vi "example 14 - splitters.vi"() -> ()   [LabVIEW 2020]
uses:
  ui-testing/ui-testing.lvlib
panel:
  out "Button clicked":string
  in  "A":bool
  in  "B":bool
  in  "C":bool
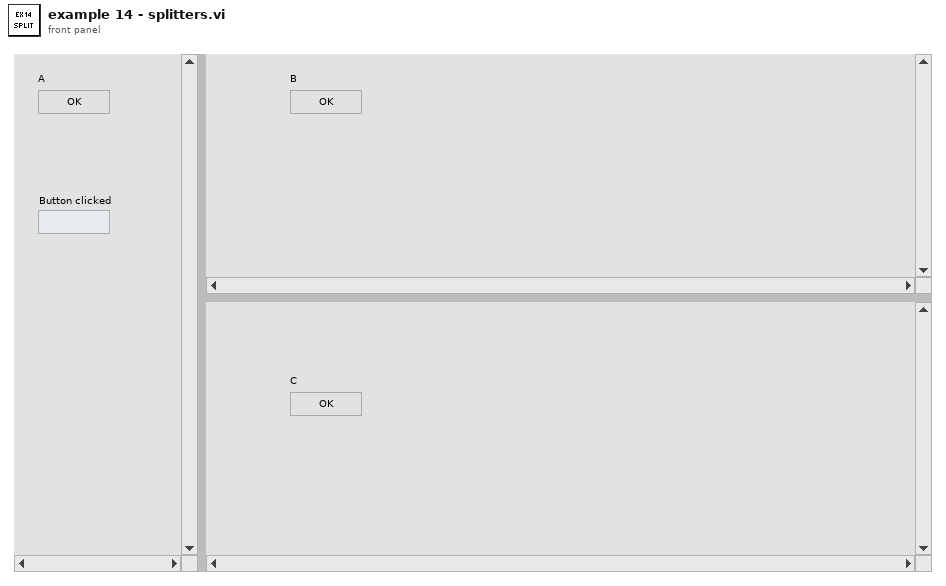
[diagram p1: front panel]
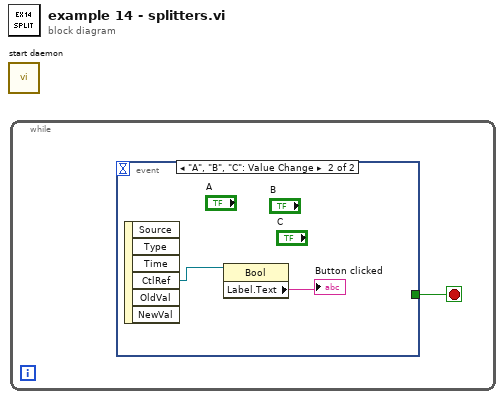
[diagram p0: block diagram]
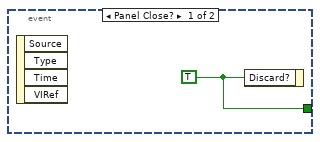
[diagram p2: hidden frame]
diagram:
  n1 = call "start daemon.vi"() -> ()  [unwired: 11 in, 1 out]
  n2 = while {
    stop <- w1 stop-if-true
    n3 = event shown="[1] \"A\", \"B\", \"C\": Value Change" {
      selector: _ -> [_ _]
      dyn-events: _ -> [_ _]
      timeout: _ -> [_ _]
      tunnel: [w2 _] -> w1
      event Panel Close? {
        w2 = TRUE
        n4 = event-data() -> ()  [unwired: 1 in, 4 out]
        n5 = event-data("Discard?"=w2) -> ()  [unwired: 1 in, 1 out]
      }
      event "A", "B", "C": Value Change {
        n6 = event-data() -> ("CtlRef"=w4:refnum<vi>)  [unwired: 1 in, 5 out]
        n7 = property class="Bool"(reference=w4) -> ("Label.Text"=→"Button clicked":string)  [unwired: 1 in, 2 out]
      }
    }
  }
